vi "Teleop DriveTwist.vi"(8 "error in":errorcluster, 9 "Deadband (pos for both)":dbl, 10 "Cap (input pos for both)":dbl, 11 "Data Input":T1) -> (0 "error out":errorcluster, 3 "Data Output":T1)   [LabVIEW 2018]
uses:
  TypeDefs/Teleop Data Cluster.ctl
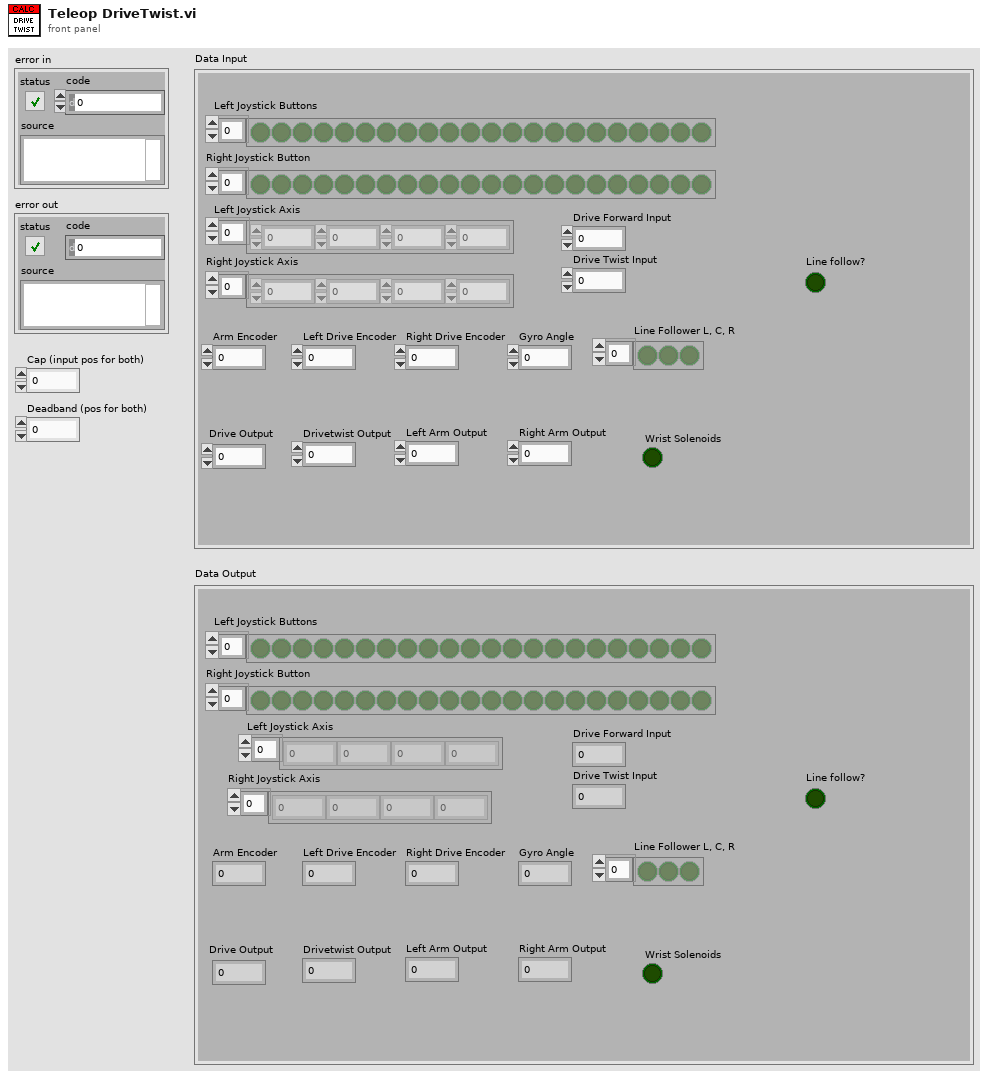
[diagram p1: front panel]
types:
  T1 = typedef "Teleop Data Cluster.ctl" = cluster{"Drive Forward Input ":dbl, "Drive Twist Input":dbl, "Drive Output":dbl, "Drivetwist Output":dbl, "Left Joystick Buttons":bool[], "Left Joystick Axis":dbl[], "Right Joystick Axis":dbl[], "Right Joystick Button":bool[], "Arm Encoder":dbl, "Left Drive Encoder":dbl, "Right Drive Encoder":dbl, "Gyro Angle ":dbl, "Left Arm Output  ":dbl, "Right Arm Output":dbl, "Line Follower L, C, R ":bool[], "Line follow?":bool, "Wrist Solenoids":bool}
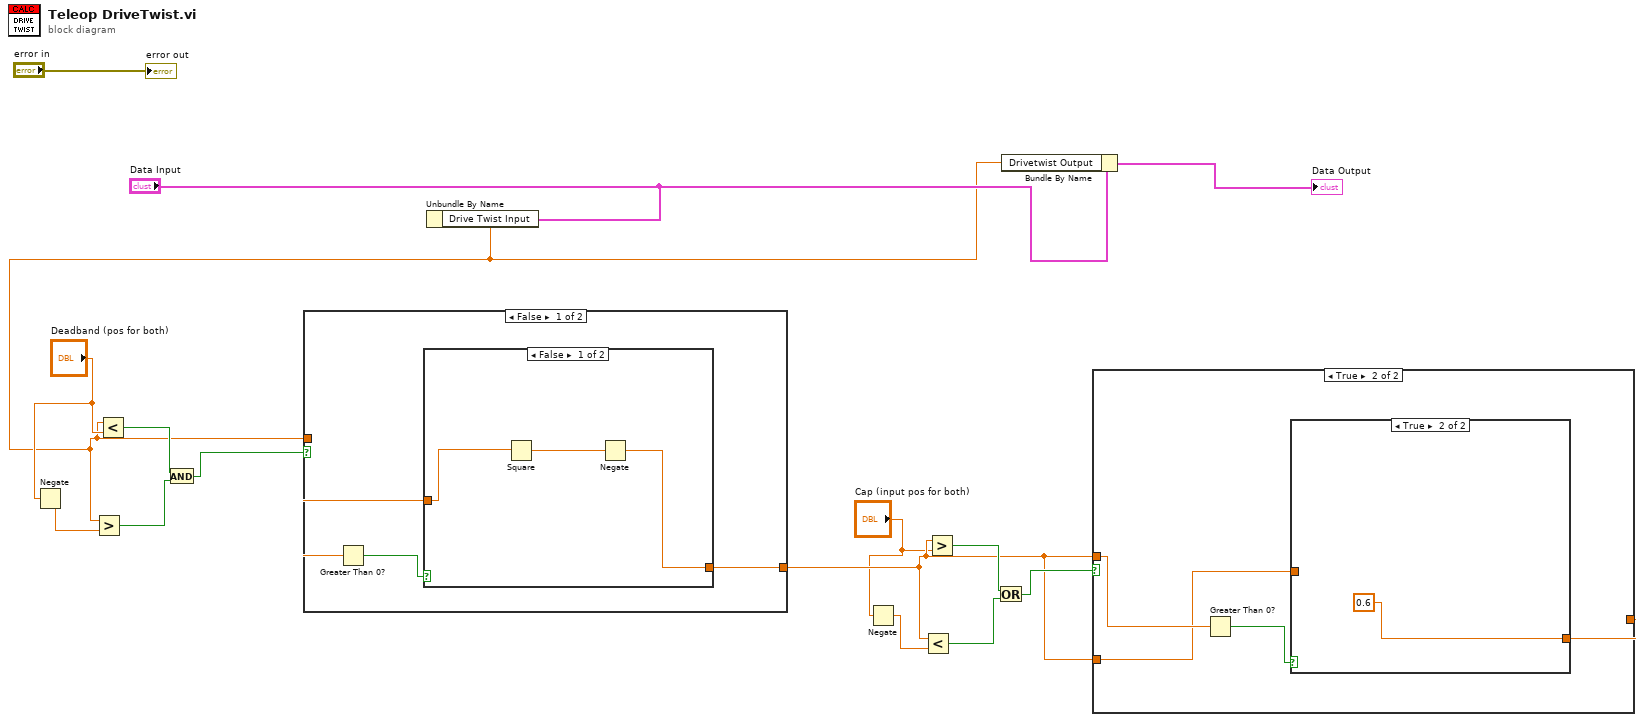
[diagram p0: block diagram]
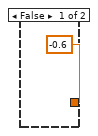
[diagram p3: hidden frame]
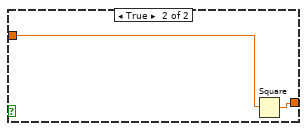
[diagram p4: hidden frame]
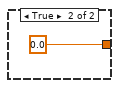
[diagram p5: hidden frame]
diagram:
  n1 = Negate(x="Deadband (pos for both)") -> (-x=w4:dbl)
  n2 = Unbundle By Name("Data Input") -> ("Drive Twist Input"=w1:dbl)
  n3 = Greater?(x=w1, y=w4) -> (0:w13:bool)
  n4 = Less?(x=w1, y="Deadband (pos for both)") -> (x < y?=w14:bool)
  n5 = And(x=w14, y=w13) -> (x .and. y?=w12:bool)
  n6 = case shown="False" w12 {
    tunnel: [w16 0.0] -> w8
    tunnel: w1 -> [w17 _]
    frame False {
      n7 = Greater Than 0?(x=w17) -> (x > 0?=w18:bool)
      n8 = case shown="False" w18 {
        tunnel: w17 -> [w20 w23]
        tunnel: [w19 w22] -> w16
        frame False {
          n9 = Square(x=w20) -> (x^2=w21:dbl)
          n10 = Negate(x=w21) -> (-x=w19:dbl)
        }
        frame True {
          n11 = Square(x=w23) -> (x^2=w22:dbl)
        }
      }
    }
    frame True {
    }
  }
  n12 = Negate(x="Cap (input pos for both)") -> (-x=w6:dbl)
  n13 = Less?(x=w8, y=w6) -> (x < y?=w10:bool)
  n14 = Greater?(x=w8, y="Cap (input pos for both)") -> (0:w11:bool)
  n15 = Or(x=w11, y=w10) -> (x .or. y?=w9:bool)
  n16 = Bundle By Name(cluster="Data Input", "Drivetwist Output"=w1) -> (→"Data Output":T1)
  n17 = case shown="True" w9 {
    tunnel: w8 -> [w25 w28]
    tunnel: [w25 w27] -> _
    tunnel: w8 -> [_ w26]
    frame False {
    }
    frame True {
      n18 = Greater Than 0?(x=w28) -> (x > 0?=w29:bool)
      n19 = case shown="True" w29 {
        tunnel: w26 -> [_ _]
        tunnel: [-0.6 0.6] -> w27
        frame False {
        }
        frame True {
        }
      }
    }
  }
  "error out" <- "error in"
